vi "Get LabVIEW Printing Settings.vi"(8 "error in (no error)":errorcluster) -> (0 "error out":errorcluster, 1 "color or monochrome":T2 items=["Unchanged", "Color/grayscale", "Monochrome"], 2 "printing method":T1 items=["Unchanged", "Standard", "PostScript", "Bitmap"], 3 "default printer name":string)   [LabVIEW 2020, in "NI_ReportGenerationCore.lvlib"]
uses:
  <vilib>/Utility/NIReport.llb/NI_ReportGenerationCore.lvlib
  <vilib>/printing/EasyPrintingControls.llb/color_or_monochrome.ctl
  <vilib>/printing/EasyPrintingControls.llb/printing_method.ctl
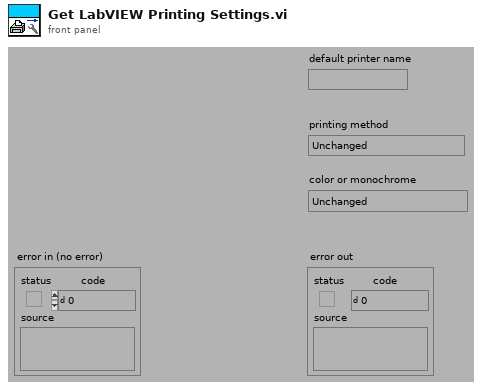
[diagram p1: front panel]
types:
  T1 = typedef "NI_ReportGenerationCore.lvlib/printing_method.ctl" = u16
  T2 = typedef "NI_ReportGenerationCore.lvlib/color_or_monochrome.ctl" = u16
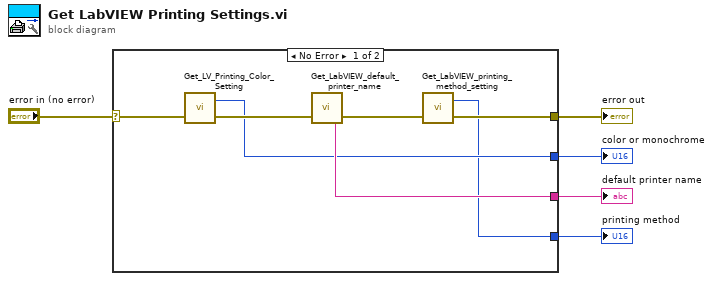
[diagram p0: block diagram]
diagram:
  n1 = case shown="No Error" "error in (no error)" {
    selector: "error in (no error)" -> [w11 w13]
    tunnel: [w7 w13] -> w4
    tunnel: [w9 _] -> w3
    tunnel: [w12 _] -> w2
    tunnel: [w6 _] -> w1
    frame No Error {
      n2 = call <vilib>:"Get_LV_Printing_Color_Setting.vi"("error in (no error)"=w11) -> ("Color?"=w9:T2, "error out"=w10:errorcluster)
      n3 = call <vilib>:"Get_LabVIEW_default_printer_name.vi"("error in (no error)"=w10) -> ("Get Default Printer"=w12:string, "error out"=w8:errorcluster)  [unwired: 2 in]
      n4 = call <vilib>:"Get_LabVIEW_printing_method_setting.vi"("error in (no error)"=w8) -> ("Print method"=w6:T1, "error out"=w7:errorcluster)
    }
    frame Error {
    }
  }
  "error out" <- w4
  "default printer name" <- w2
  "printing method" <- w1
  "color or monochrome" <- w3
